vi "$IO_18V7TankControl.vi"(6 "error in":errorcluster, 7 "VISA Refnum in":refnum<visa-resource-name>="COM5", 8 "Pump Params":T1={"Empty Inches"=8.4, "Full Inches"=2.75, "RNG_SLOW"=0.5, "RNG_CREEP"=0.007, "RNG_STOP "=0.002, "VISA resource name"="Default", "SPD_SLOW"=30, "SPD_CREEP"=7, "SPD_FAST"=100, "Zero template"=path "30", "zero  Settle sec"=5, "Laser Slope"=-0.996, "Laser Offset"=9.601, "Sim Fill Rate"=4000.0, "Cal Date"="1/26/2024", "Cal Technician"="Default"} {"Sim Fill Rate" format="%.3f"; "Laser Offset" format="%.3f"; "Laser Slope" format="%.3f"; "RNG_STOP" format="%#_13g"; "RNG_CREEP" format="%#_13g"; "RNG_SLOW" format="%#_13g"}, 9 "Speed":i16, 10 "Fill!Drain":bool, 11 "Raw/!Saled Level":bool) -> (1 "Level PV":sgl=9.601, 2 "Level":cluster{"Laser Raw":sgl, "Laser Scaled":dbl}={"Laser Raw"=0.0, "Laser Scaled"=9.60099983215332} {"Laser Scaled" scale=0.0..10.0}, 4 "error out":errorcluster, 5 "VISA Refnum out":refnum<visa-resource-name>="COM5")   [LabVIEW 2024]
uses:
  Control Definitions/DEF_PumpParams.ctl
  Keyance Demo Code/Keyence LK-G3000/Keyence LK-G3000.lvlib
panel:
  out "TX Buf":string="D0\r"
  out "read buffer ASC":string
  # "Use this Timer section\nto measure the Level dl/dt"
  # "Use if off line to generate\na test Reply to Write msg"
  # "Target Speed for PWC OLS = 0.52\"/min\nWhich is Speed set to ~17% which 24Vdc"
  # "Laser ON When Laser\nis on Line."
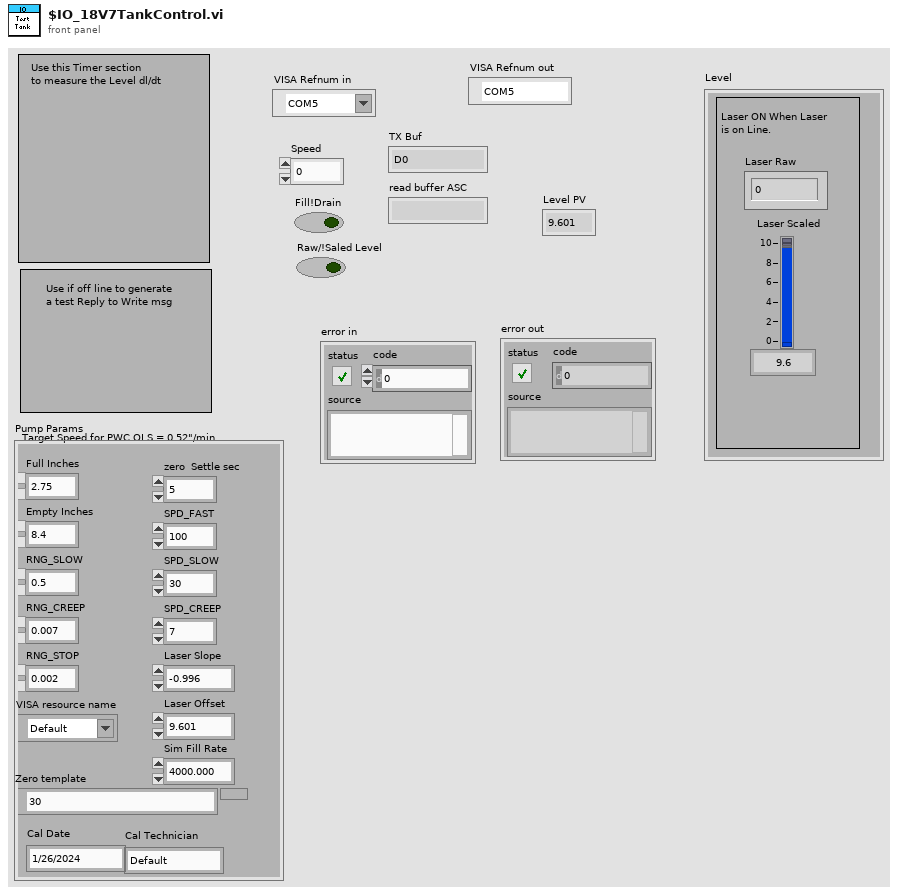
[diagram p1: front panel]
types:
  T1 = typedef "DEF_PumpParams.ctl" = cluster{"Empty Inches":dbl, "Full Inches":dbl, "RNG_SLOW":dbl, "RNG_CREEP":dbl, "RNG_STOP ":dbl, "VISA resource name":refnum<visa-resource-name>, "SPD_SLOW":i32, "SPD_CREEP":i32, "SPD_FAST":i32, "Zero template":path, "zero  Settle sec":i32, "Laser Slope":sgl, "Laser Offset":sgl, "Sim Fill Rate":sgl, "Cal Date":string, "Cal Technician":string}
  T2 = cluster{"Fill!Drain":bool, "Speed":i16, "Send Msg":bool, "Write Buf":string}
  T3 = typedef "Keyence LK-G3000.lvlib/LKIF_FLOATVALUE.ctl" = cluster{"LKIF_FLOATRESULT":T4, "Value":sgl}
  T4 = typedef "Keyence LK-G3000.lvlib/LKIF_FLOATRESULT.ctl" = i32
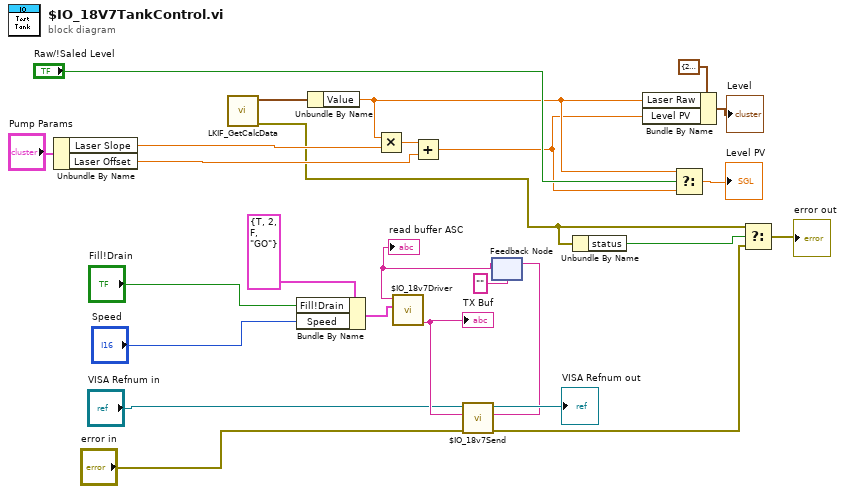
[diagram p0: block diagram]
diagram:
  n1 = Unbundle By Name("Pump Params") -> ("Laser Slope"=w11:sgl, "Laser Offset"=w10:sgl)
  n2 = call "LKIF_GetCalcData.vi"() -> ("error out"=w1:errorcluster, "CalcData1"=w2:T3)  [unwired: 9 in, 1 out]
  n3 = Bundle By Name(cluster=T2 {"Fill!Drain"=TRUE, "Speed"=2, "Send Msg"=FALSE, "Write Buf"="GO"} ("Inputs"), "Fill!Drain"="Fill!Drain", "Speed"="Speed") -> (w23:T2)
  n4 = Unbundle By Name(w2) -> ("Value"=w4:sgl)
  n5 = Multiply(x=w4, y=w11) -> (x*y=w8:sgl)
  n6 = Add(x=w8, y=w10) -> (x+y=w3:sgl)
  n7 = feedback #1("" ("read buffer")) -> (w17:string)
  "read buffer ASC" <- w17
  n8 = call "$IO_18v7Driver.vi"("Inputs"=w23, "Reply In"=w17) -> ("Tx Buf Out"=w25:string)  [unwired: 8 in, 1 out]
  "TX Buf" <- w25
  n9 = call "$IO_18v7Send.vi"("error in (no error)"="error in", "Tx Buf Out"=w25, "VISA Refnum in"="VISA Refnum in") -> ("error out"=w15:errorcluster, "read buffer"=w18:string, "VISA Refnum out"=→"VISA Refnum out":refnum<visa-resource-name>)  [unwired: 6 in]
  n10 = feedback-in #1(w18) -> ()
  n11 = Unbundle By Name(w1) -> ("status"=w13:bool)
  n12 = Bundle By Name(cluster=cluster{"Laser Raw":sgl, "Level PV":dbl} {"Laser Raw"=2.4953, "Level PV"=7.1220598220825195} ("Level"), "Laser Raw"=w4, "Level PV"=w3) -> (→"Level":cluster{"Laser Raw":sgl, "Level PV":dbl})
  n13 = Select(t=w4, s="Raw/!Saled Level", f=w3) -> (s? t:f=→"Level PV":sgl)
  n14 = Select(t=w1, s=w13, f=w15) -> (s? t:f=→"error out":errorcluster)
